vi "Unevenly_spaced_spectra_ph.vi"(2 "Current Block No":i32, 3 "Shift in":dbl[](array[numeric]), 4 "U":dbl[](array[numeric]), 5 "Time":dbl[](array[numeric])) -> (0 "Sum E(F)":dbl[](array[numeric]), 1 "Freq":dbl[](array[numeric]))   [LabVIEW 2010]
uses:
  <vilib>/gmath/NI_Gmath.lvlib
panel:
  out "XY Graph 2":cluster{"Freq":dbl[], dbl[]}[](graph)
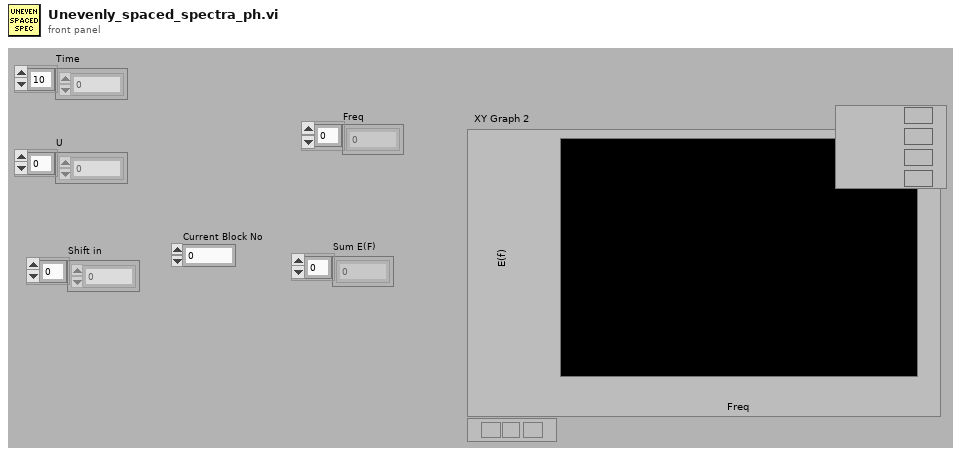
[diagram p1: front panel]
types:
  T1 = cluster{"Power Spectrum FFT {X} Frequency":dbl[], "Power Spectrum FFT {X}":dbl[]}
  T2 = cluster{"Power Spectrum FFT {X} Frequency":dbl[], "Power Spectrum FFT {X}":dbl[]}[]
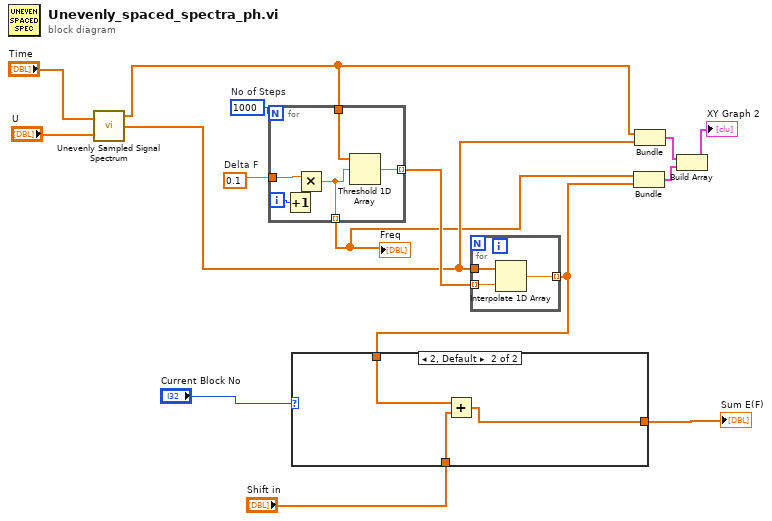
[diagram p0: block diagram]
diagram:
  w11 = 0.1  # Delta F
  w12 = 1000  # No of Steps
  n1 = call <vilib>:"Unevenly Sampled Signal Spectrum.vi"("XTime"="Time", "X"="U") -> ("Power Spectrum FFT {X} Frequency"=w7:dbl[], "Power Spectrum FFT {X}"=w6:dbl[])  [unwired: 1 out]
  n2 = for {
    N: w12 -> [_]
    tunnel: w11 -> [w20]
    tunnel: w7 -> [w19]
    tunnel: [w18] -> w13 mode=indexing
    tunnel: [w17] -> w5 mode=indexing
    i -> [w21]
    n3 = Increment(x=w21) -> (x+1=w16:i32)
    n4 = Multiply(x=w20, y=w16) -> (x*y=w17:dbl)
    n5 = Threshold 1D Array(2:w17, 3:w19) -> (0:w18:dbl)  [unwired: 1 out]
  }
  "Freq" <- w5
  n6 = for {
    tunnel: w6 -> [w24]
    tunnel: w13 -> [w23] mode=indexing
    tunnel: [w22] -> w4 mode=indexing
    n7 = Interpolate 1D Array(1:w23, 2:w24) -> (0:w22:dbl)
  }
  n8 = case shown="2, Default" "Current Block No" {
    tunnel: [w25 w26] -> w10
    tunnel: w4 -> [w25 w28]
    tunnel: "Shift in" -> [_ w27]
    frame 1 {
    }
    frame 2, Default {
      n9 = Add(x=w28, y=w27) -> (x+y=w26:dbl[])
    }
  }
  "Sum E(F)" <- w10
  n10 = Bundle(w5, w4) -> (w2:cluster{dbl[], dbl[]})  [unwired: 1 in]
  n11 = Bundle("Power Spectrum FFT {X} Frequency"=w7, "Power Spectrum FFT {X}"=w6) -> (w3:T1)  [unwired: 1 in]
  n12 = Build Array(w3, w2) -> (→"XY Graph 2":T2)
